vi "Dashboard Main.vi"() -> ()   [LabVIEW 2015]
uses:
  <vilib>/Rock Robotics/WPI/CAN/TalonSRX/WPI_CANTalonSRX_ControlMode.ctl
  <vilib>/Utility/miscctls.llb/LVRowAndColumnTypeDef.ctl
  <vilib>/event_ctls.llb/eventvkey.ctl
  <vilib>/Rock Robotics/WPI/Dashboard/WPI_DashboardLogging Global.vi
  <vilib>/Rock Robotics/Network Tables/NT Read Numeric Array.vi
  <vilib>/Utility/config.llb/Write Key (String).vi
  <vilib>/Utility/config.llb/Write Key (I32).vi
  <vilib>/Utility/config.llb/NI_LVConfig.lvlib
panel:
  in  "Arm State":enum16{"Up", "Down"}(ring)=enum."Down"
  in  "TCP":refnum<k5>
  out "Camera IP":string
  out "Image Message":string="Timeout in Camera Communications"
  in  "Dashboard Tab":T1(tab)
  out "PhotoEye":bool
  in  "Raw Speed":dbl
  out "READY":bool
  out "Shooter Speed":dbl(knob) scale=0.0..100.0
  out "Target Distance":dbl(slide) scale=0.0..30.0
  out "Target Acquired":bool
  in  "Select Auto":string(combo)
  out "NT Connection":bool
  in  "Camera Settings":T2={"Frame Rate"=30, "Compression"=30, "Size"=1} {"Frame Rate" scale=1.0..30.0; "Size" items=["640x480", "320x240", "160x120"]}
  out "MotorChart R":cluster{"Numeric":dbl, "Numeric":dbl}(graph)
  out "MotorChart L":T3(graph)
  out "MotorSliders R":cluster{"MotorSlide1":dbl, "MotorSlide2":dbl} {"MotorSlide2" scale=-1.0..1.0 scale format="%#_2e"; "MotorSlide1" scale=-1.0..1.0 scale format="%#_2e"}
  out "MotorSliders L":T4 {"MotorSlide4 2" scale=0.0..14.0 scale format="%#_2e"; "MotorSlide2" scale=-1.0..1.0 scale format="%#_2e"; "MotorSlide1" scale=-1.0..1.0 scale format="%#_2e"}
  out "JS1 Z":dbl(slide) scale=-1.0..1.0 scale format="%#_2e"
  out "JS1 Graph":cluster{"X":dbl, "Y":dbl}[](graph)
  out "JS1 Buttons":T5
  out "JS2 Z":dbl(slide) scale=-1.0..1.0 scale format="%#_2e"
  out "JS2 Graph":cluster{"X":dbl, "Y":dbl}[](graph)
  out "JS2 Buttons":T5
  out "Mode":T6(ring)=enum."Auto Disabled"
  in  "DB Camera Config":bool
  out "fps":dbl format="%#.1g"
  out "Mbps":dbl format="%#.1g"
  out "Mbps LED":bool
  out "Arm Down":bool
  out "Arm Up":bool
  in  "Vision":u16(ring) items=["Camera Off", "USB Camera SW", "USB Camera HW", "IP Camera"]
  in  "Rec Mode":enum32{"Stop", "Record", "Playback"}(radio)
  out "AUTO 4":bool
  out "AUTO 2":bool
  out "AUTO 1":bool
  out "NO AUTO":bool
  in  "Select Autonomous":u16(knob) scale=0.0..4.0
  out "AUTO 3":bool
  in  "Talon SRX Mode":T7
  in  "Test Slider":dbl(slide) scale=0.0..100.0 scale format="%#_3g"
  in  "On/Off":bool caption="Solenoid"
  in  "Test Name":u16(ring) items=["Select the test to run..."]
  in  "Test Tree":string(tree)
  in  "Motor":cluster{"Value":dbl, "Enable":bool} {"Value" scale=-1.0..1.0 scale format="%#_3g"}
  out "Progress":T8 {"Test Progress" scale=0.0..100.0}
  in  "Rev/Fwd":cluster{"Forward":bool, "Reverse":bool}
  in  "Test Ring":u16(ring) items=["Monochrome", "Color"]
  out "Cmd Status":string
  in  "Execute Command":bool
  in  "Command Params":string[][](table)
  in  "Command Selection":i32(listbox)
  in  "CheckList":i32(listbox)
  out "Tree":string(tree)
  out "Camera Image":T9(plugin-control)
  out "Background":bool
  # "Left"
  # "Front"
  # "Right"
  # "Battery"
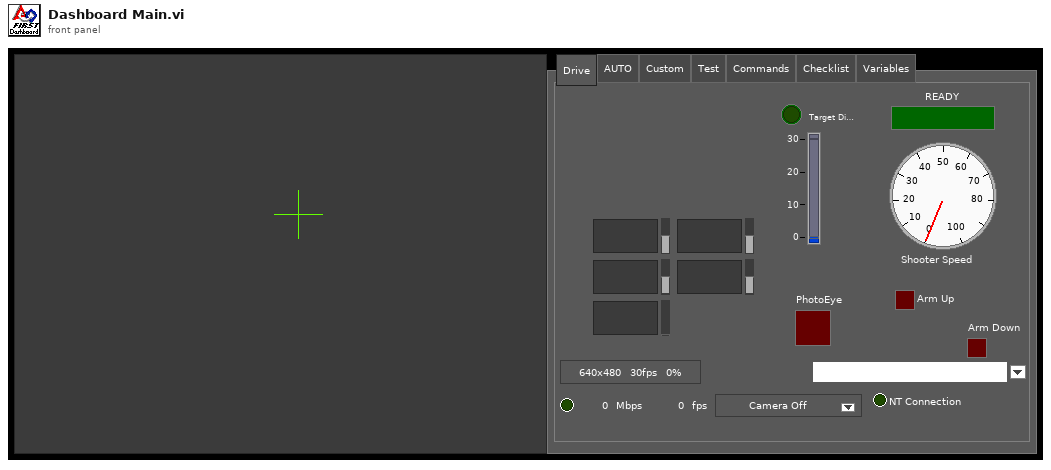
[diagram p1: front panel]
types:
  T1 = enum32{"Drive", "AUTO", "Custom", "Test", "Commands", "Checklist", "Variables"}
  T2 = cluster{"Frame Rate":i32, "Compression":i32, "Size":u16}
  T3 = cluster{"Numeric":dbl, "Numeric":dbl, "Battery V":dbl}
  T4 = cluster{"MotorSlide1":dbl, "MotorSlide2":dbl, "MotorSlide4 2":dbl}
  T5 = cluster{bool, bool, bool, bool, bool, bool, bool, bool, bool, bool, bool, bool}
  T6 = enum8{"Tele-Op Disabled", "Tele-Op Enabled", "Auto Disabled", "Auto Enabled", "Test Disabled", "Test Enabled", "Disconnected", "No Code", "E-Stop"}
  T7 = typedef "WPI_CANTalonSRX_ControlMode.ctl" = enum16{"Throttle (Duty-Cycle)", "Position Closed-Loop", "Velocity Closed-Loop", "Current Closed-Loop", "Voltage Compensation", "Slave Follower", "Motion Profile"}
  T8 = cluster{"Test Progress":u8, "Test Progress Text":string}
  T9 = typedef "IMAQ Image.ctl" = refnum<image>
  T10 = cluster{"IDs":cluster{"RPC field ID":u16, "Unique ID":u16}, "String":string}
  T11 = enum32{"Drive", "Basic", "AUTO", "Test", "Checklist", "Variables"}
  T12 = enum32{"Drive", "Basic", "Custom", "Test", "Checklist", "Variables"}
  T13 = typedef "Image Type" = u32
  T14 = cluster{"Error Strings":string, "Disable Counts":cluster{u16, u16}, "Rail Faults":cluster{u16, u16, u16}, "Robot IP":string, "DB Mode":u8, "Event Info":cluster{"Name":string, "Type":u8, "Number":u16, "Replay":u8}, "Camera Addr":string}
  T15 = cluster{"Storage":cluster{"Disk Free":u64, "RAM Block":u32, "RAM free":u32}, "CPU Utilization":cluster{"CPU % ISR":sgl, "CPU % Time Crit":sgl, "CPU % Timed Str":sgl, "CPU % High":sgl, "CPU % Above":sgl, "CPU % Normal":sgl, "CPU % Low":sgl}, "CAN":cluster{"% Bus Utilization":sgl, "Bus Off Cnt":u32, "TX_FIFO Full Cnt":u32, "Receive Error Cnt":u8, "Transmit Error Cnt":u8}, "HID":cluster{"HID Outputs":u32, "Rumble Low":u16, "Rumble High":u16}[]}
  T16 = cluster{"Status bits":cluster{"Test Mode":bool, "Autonomous":bool, "Enabled":bool, "Code Start":bool, "Brownout":bool, "Reserved 2":bool, "Reserved 3":bool, "E-Stop":bool}, "Code Trace":cluster{"Disabled":bool, "TeleOp":bool, "Auto":bool, "Test":bool}, "Controller Type":enum16{"unknown", "cRIO", "roboRio"}, "Code?":enum16{"unknown", "noCode", "code"}, "Battery V":dbl}
  T17 = cluster{"Control Bits":cluster{"TestMode":bool, "Autonomous":bool, "Enabled":bool, "FMS Present":bool, bool, bool, bool, "E-Stop":bool}, "Team Station ":u8, "Countdown":sgl, "Joystick Values":cluster{"Axes":dbl[], "Buttons":bool[], "POVs":i16[]}[]}
  T18 = cluster{"Axes":dbl[], "Buttons":bool[], "POVs":i16[]}[]
  T19 = cluster{"Axes":dbl[], "Buttons":bool[], "POVs":i16[]}
  T20 = cluster{"Buttons[0]":bool, "Buttons[1]":bool, "Buttons[2]":bool, "Buttons[3]":bool, "Buttons[4]":bool, "Buttons[5]":bool, "Buttons[6]":bool, "Buttons[7]":bool, "Buttons[8]":bool, "Buttons[9]":bool, "Buttons[10]":bool, "Buttons[11]":bool}
  T21 = typedef "NI_LVConfig.lvlib/Config Data RefNum.ctl" = refnum<k1>
  T22 = cluster{"Operation":enum16{"Update", "Clear"}, "Color Box":u32}[]
  T23 = typedef "eventvkey.ctl" = enum16{"ASCII", "Enter", "Return", "Shift", "Ctrl", "Alt", "Cmd", "Opt", "Caps", "NumLock", "Clear", "Break", "Up", "Down", "Left", "Right", "Insert", "Delete", "Home", "End", "PageUp", "PageDown", "Escape", "Help", "Pause", "ScrollLock", "F1", "F2", "F3", "F4", "F5", "F6", "F7", "F8", "F9", "F10", "F11", "F12", "F13", "F14", "F15", "F16", "F17", "F18", "F19", "F20", "F21", "F22", "F23", "F24", "Play", "VolumeUp", "VolumeDown", "Mute", "Two Byte Char"}
  T24 = cluster{"Image Size":bool, "Image Type":bool, "Pixel Value":bool, "ROI Information":bool, "Zoom Factor":bool}
  T25 = enum8{"Enabled", "Disabled", "Disabled and Grayed Out"}
  T26 = cluster{"Operation":enum16{"Update", "Clear"}, "Color Box":u32}
  T27 = typedef "LVRowAndColumnTypeDef.ctl" = cluster{"Row":i32, "Column":i32}
  T28 = cluster{"Shift":bool, "Ctrl":bool, "Alt":bool, "Cmd":bool, "Opt":bool}
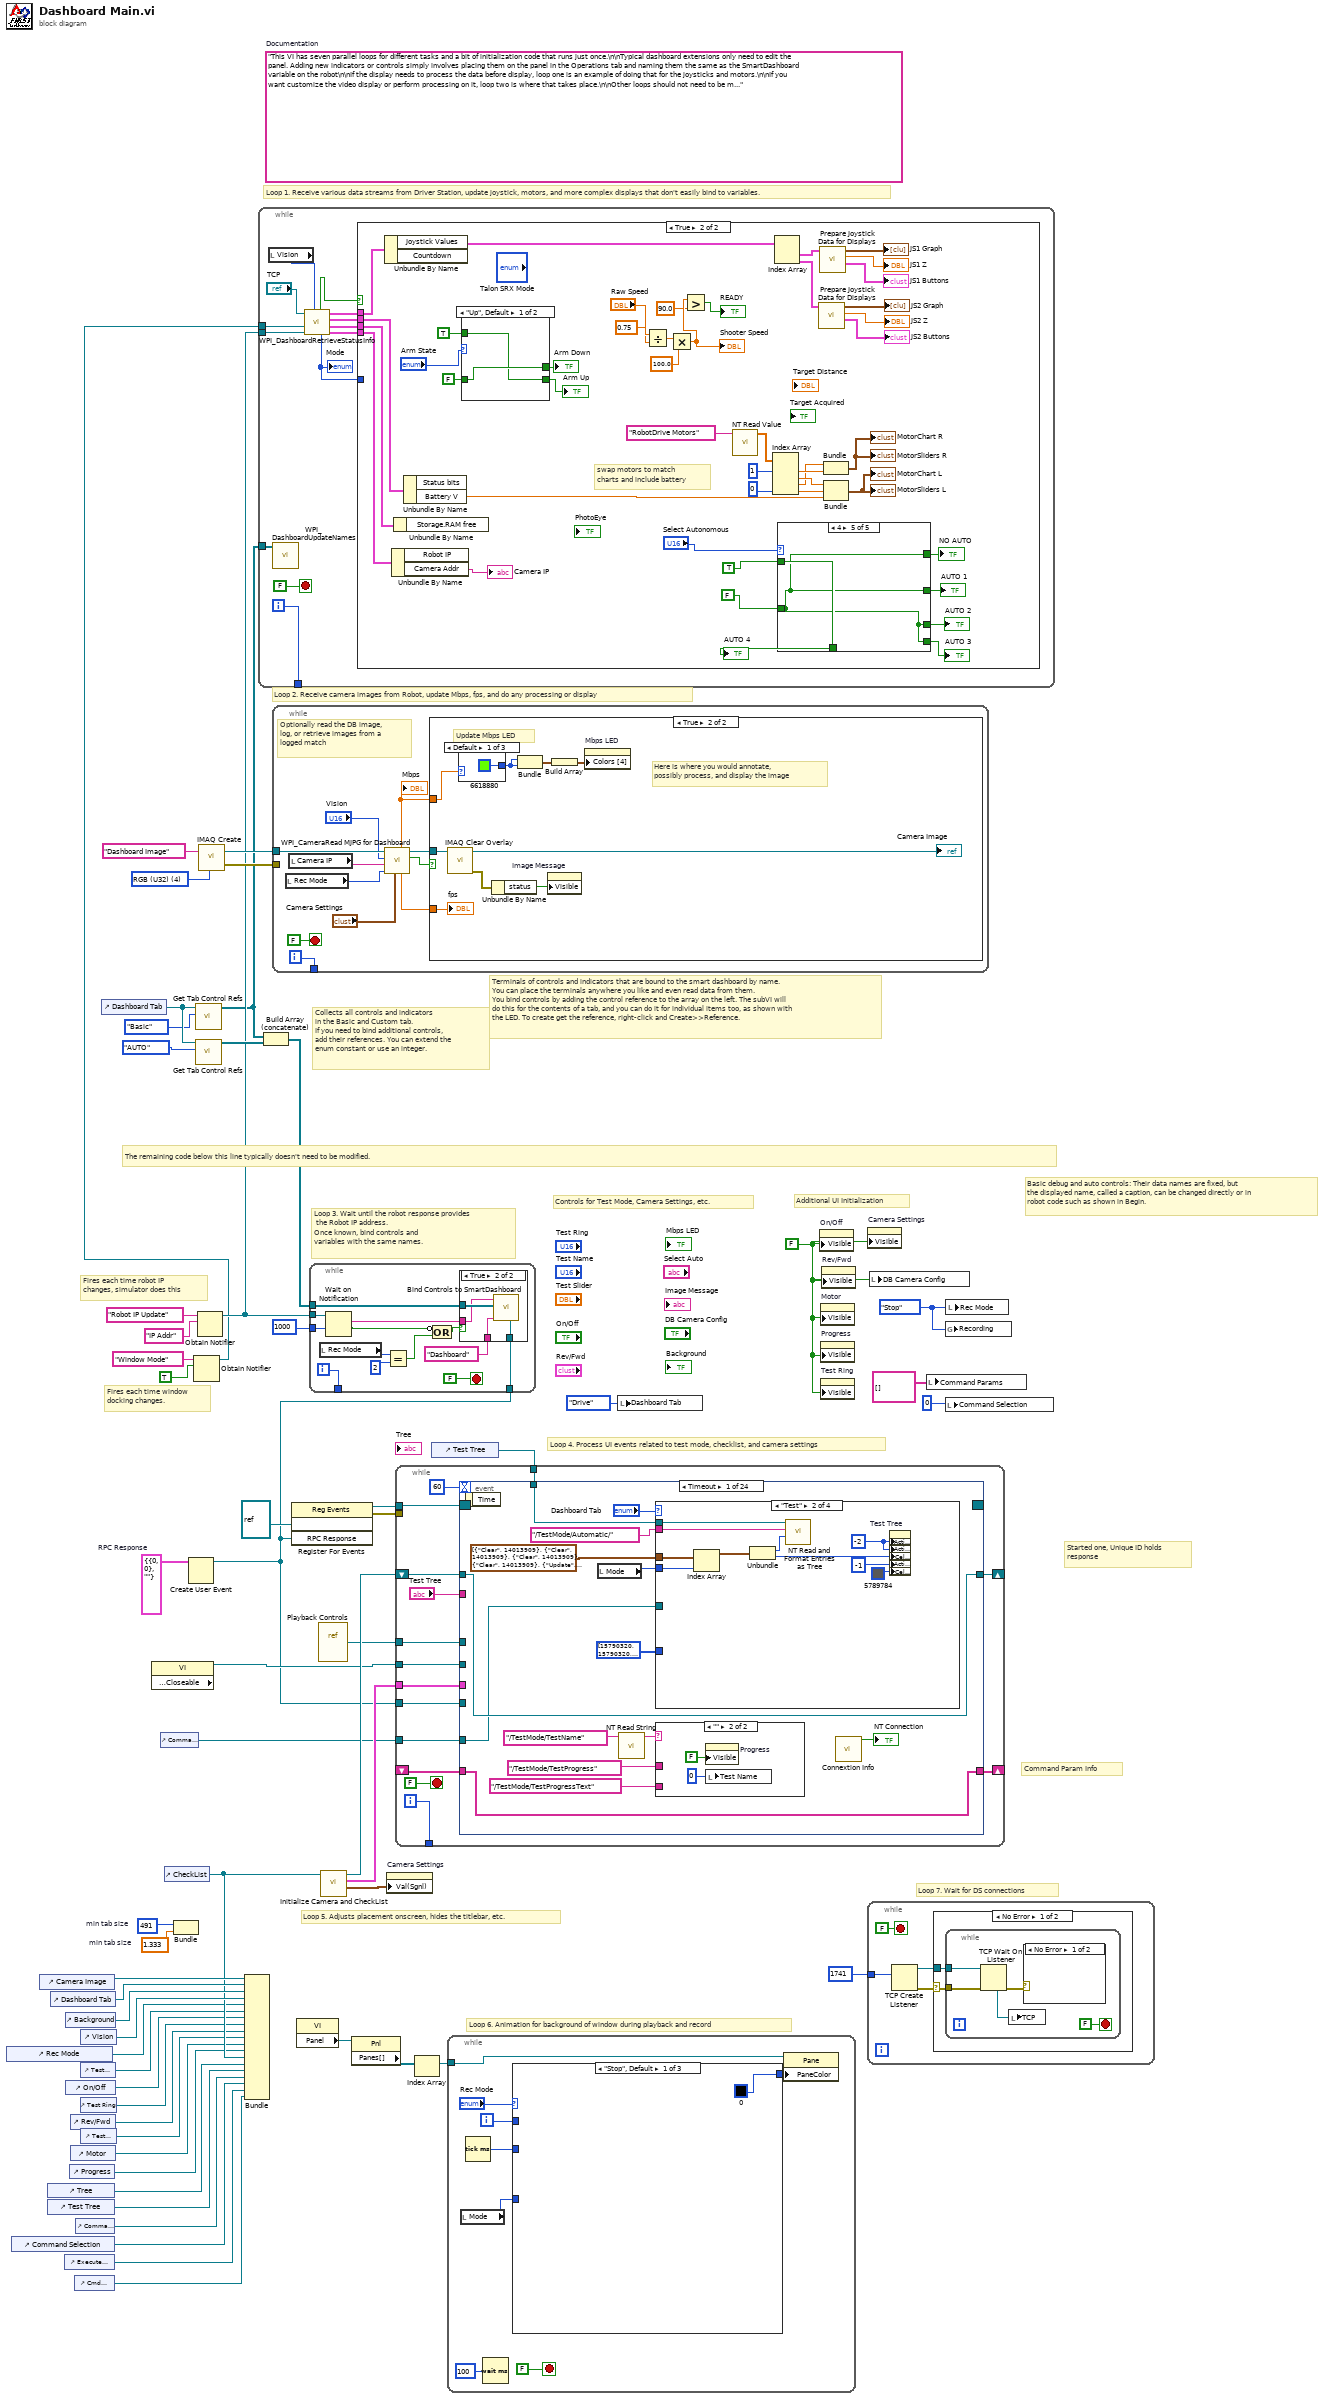
[diagram p0: block diagram]
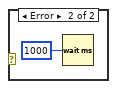
[diagram p2: hidden frame]
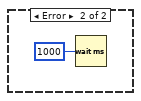
[diagram p3: hidden frame]
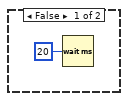
[diagram p4: hidden frame]
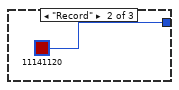
[diagram p10: hidden frame]
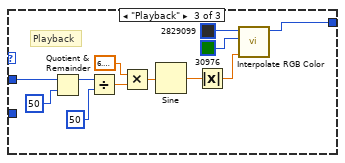
[diagram p11: hidden frame]
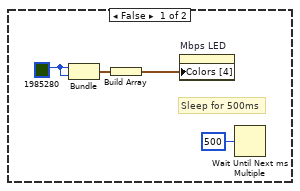
[diagram p13: hidden frame]
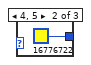
[diagram p14: hidden frame]
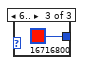
[diagram p15: hidden frame]
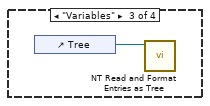
[diagram p17: hidden frame]
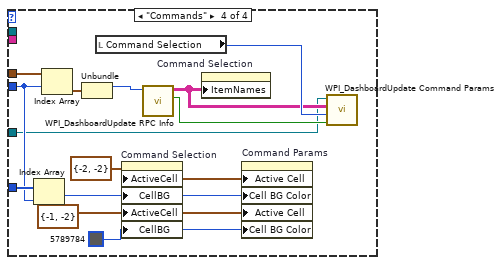
[diagram p18: hidden frame]
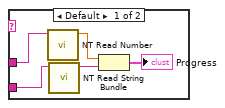
[diagram p19: hidden frame]
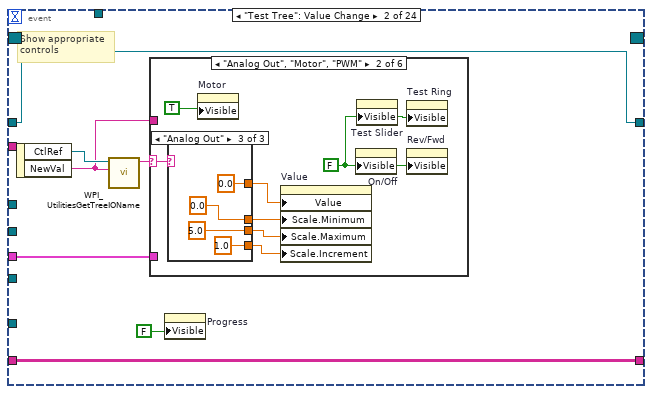
[diagram p20: hidden frame]
diagram:
  w8 = T10 {"IDs"={"RPC field ID"=0, "Unique ID"=0}, "String"=""}  # RPC Response
  w31 = 491  # min tab size
  w30 = 1.333  # min tab size
  w39 = enum32{"Stop", "Record", "Playback"}."Stop" ("Rec Mode")
  w15 = FALSE ("Visible")
  (unwired) "This VI has seven parallel loops for different tasks and a bit of initialization code that runs just once.\n\nTypical dashboard extensions only need to edit the panel. Adding new indicators or controls simply involves placing them on the panel in the Operations tab and naming them the same as the SmartDashboard variable on the robot\n\nIf the display needs to process the data before display, loop one is an example of doing that for the joysticks and motors.\n\nIf you want customize the video display or perform processing on it, loop two is where that takes place.\n\nOther loops should not need to be modified. They are pretty standard, and document the task they perform."  # Documentation
  w59 = T13 4 items=["Grayscale (U8)", "Grayscale (I16)", "Grayscale (SGL)", "Complex (CSG)", "RGB (U32)", "HSL (U32)", "RGB (U64)"] ("Image Type")
  # "Command Param Info"
  # "Started one, Unique ID holds\nresponse"
  # "Loop 7. Wait for DS connections"
  # "Basic debug and auto controls: Their data names are fixed, but\nthe displayed name, called a caption, can be changed directly or in\nrobot code such as shown in Begin."
  # "Controls for Test Mode, Camera Settings, etc."
  # "Additional UI Initialization"
  # "Loop 6. Animation for background of window during playback and record"
  # "Fires each time robot IP\nchanges, simulator does this"
  # "Fires each time window\ndocking changes."
  # "Collects all controls and indicators\nin the Basic and Custom tab.\nIf you need to bind additional controls,\nadd their references. You can extend the\nenum constant or use an integer."
  # "The remaining code below this line typically doesn't need to be modified."
  # "Loop 4. Process UI events related to test mode, checklist, and camera settings"
  # "Terminals of controls and indicators that are bound to the smart dashboard by name.\nYou can place the terminals anywhere you like and even read data from them.\nYou bind controls by adding the control reference to the array on the left. The subVI will\ndo this for the contents of a tab, and you can do it for individual items too, as shown with\nthe LED. To create get the reference, right-click and Create>>Reference."
  # "Loop 3. Wait until the robot response provides\n the Robot IP address.\nOnce known, bind controls and\nvariables with the same names."
  # "Loop 5. Adjusts placement onscreen, hides the titlebar, etc."
  # "Loop 1. Receive various data streams from Driver Station, update joystick, motors, and more complex displays that don't easily bind to variables."
  # "Loop 2. Receive camera images from Robot, update Mbps, fps, and do any processing or display"
  n1 = control-ref of="Rec Mode"() -> (w21:refnum<vi>)
  n2 = control-ref of="Command Selection"() -> (w7:refnum<vi>)
  n3 = control-ref of="Camera Image"() -> (w34:refnum<vi>)
  n4 = control-ref of="Tree"() -> (w25:refnum<vi>)
  n5 = control-ref of="Test Tree"() -> (w24:refnum<vi>)
  n6 = control-ref of="Dashboard Tab"() -> (w33:refnum<vi>)
  n7 = control-ref of="Execute Command"() -> (w9:refnum<vi>)
  n8 = control-ref of="Background"() -> (w29:refnum<vi>)
  n9 = control-ref of="On/Off"() -> (w19:refnum<vi>)
  n10 = control-ref of="Progress"() -> (w16:refnum<vi>)
  n11 = control-ref of="Rev/Fwd"() -> (w17:refnum<vi>)
  n12 = control-ref of="Motor"() -> (w22:refnum<vi>)
  n13 = control-ref of="Cmd Status"() -> (w3:refnum<vi>)
  n14 = control-ref of="Command Params"() -> (w10:refnum<vi>)
  n15 = control-ref of="Test Slider"() -> (w20:refnum<vi>)
  n16 = control-ref of="Vision"() -> (w32:refnum<vi>)
  n17 = control-ref of="Test Ring"() -> (w18:refnum<vi>)
  n18 = control-ref of="Test Name"() -> (w23:refnum<vi>)
  n19 = control-ref of="Dashboard Tab"() -> (w37:refnum<vi>)
  n20 = property class="VI" props=["Front Panel.Closeable"]() -> (reference out=w38:refnum<vi>)  [unwired: 2 in, 2 out]
  n21 = control-ref of="Command Params"() -> (w2:refnum<vi>)
  n22 = control-ref of="CheckList"() -> (w26:refnum<vi>)
  n23 = Bundle("min tab size"=w31, "min tab size"=w30) -> ()  [unwired: 1 in, 1 out]
  n24 = Create User Event(user event datatype=w8) -> (user event=w4:refnum<user-event>)  [unwired: 1 in, 1 out]
  n25 = Obtain Notifier(name (unnamed)="Window Mode", notification data type=TRUE) -> (notifier out=w12:refnum<notifier>)  [unwired: 2 in, 2 out]
  n26 = call <vilib>:"Get Tab Control Refs.vi"("Page Index"=T12."Basic" ("Dashboard Tab"), "TabControl in"=w37) -> ("ControlsOnPage"=w13:refnum<vi>[])  [unwired: 9 in]
  n27 = call <vilib>:"Get Tab Control Refs.vi"("Page Index"=T11."AUTO" ("Dashboard Tab"), "TabControl in"=w37) -> ("ControlsOnPage"=w36:refnum<vi>[])  [unwired: 9 in]
  n28 = Obtain Notifier(name (unnamed)="Robot IP Update", notification data type="IP Addr" ("name (unnamed)")) -> (notifier out=w14:refnum<notifier>)  [unwired: 2 in, 2 out]
  n29 = call "IMAQ Create"("Image Name"="Dashboard Image", "Image Type"=w59) -> ("New Image"=w57:T9, "error out"=w56:errorcluster)  [unwired: 2 in, 1 out]
  n30 = Bundle("Camera Image"=w34, "Dashboard Tab"=w33, "Background"=w29, "Vision"=w32, "Rec Mode"=w21, "Test Slider"=w20, "On/Off"=w19, "Test Ring"=w18, "Rev/Fwd"=w17, "Test Name"=w23, "Motor"=w22, "Progress"=w16, "CheckList"=w26, "Tree"=w25, "Test Tree"=w24, "Command Params"=w10, "Command Selection"=w7, "Execute Command"=w9, "Cmd Status"=w3) -> ()  [unwired: 1 in, 1 out]
  n31 = while {
    tunnel: [w71] -> _
    tunnel: w14 -> [w66]
    tunnel: w13 -> [w65]
    tunnel: w12 -> [w61]
    i -> [w71]
    stop <- FALSE stop-if-true
    n32 = local read "Vision"() -> (w63:u16)
    n33 = call <vilib>:"WPI_DashboardUpdateNames.vi"("Controls on Tab"=w65) -> ()  [unwired: 11 in]
    n34 = call <vilib>:"WPI_DashboardRetrieveStatusInfo.vi"("Vision"=w63, "Binding Refnum"=w66, "Window Mode Notifier"=w61, "TCP Cnx"="TCP") -> ("Power and Errors"=w67:T14, "Robot Metrics"=w69:T15, "Status Info"=w70:T16, "Control Info"=w68:T17, "Robot Mode"=w64:T6, "Process?"=w60:bool)  [unwired: 2 in]
    "Mode" <- w64
    n35 = case shown="True" w60 {
      tunnel: w70 -> [_ w118]
      tunnel: w69 -> [_ w117]
      tunnel: w68 -> [_ w116]
      tunnel: w67 -> [_ w115]
      tunnel: w64 -> [_ _]
      frame False {
        n36 = Wait (ms)(milliseconds to wait=u32 20) -> ()  [unwired: 1 out]
      }
      frame True {
        # "swap motors to match\ncharts and include battery"
        n37 = Unbundle By Name(w116) -> ("Joystick Values"=w105:T18)  [unwired: 1 out]
        n38 = Unbundle By Name(w115) -> ("Camera Addr"=→"Camera IP":string)  [unwired: 1 out]
        n39 = Unbundle By Name(w117) -> ()  [unwired: 1 out]
        n40 = Unbundle By Name(w118) -> ("Battery V"=w106:dbl)  [unwired: 1 out]
        n41 = case shown="\"Up\", Default" "Arm State" {
          tunnel: TRUE -> [w119 w122]
          tunnel: FALSE -> [w120 w121]
          tunnel: [w120 w122] -> w81
          tunnel: [w119 w121] -> w80
          frame "Up", Default {
          }
          frame "Down" {
          }
        }
        "Arm Down" <- w81
        "Arm Up" <- w80
        n42 = Divide(x="Raw Speed", y=0.75) -> (x/y=w91:dbl)
        n43 = Multiply(x=w91, y=100.0) -> (x*y=w88:dbl)
        "Shooter Speed" <- w88
        n44 = Greater?(x=w88, y=90.0) -> (0:→"READY":bool)
        n45 = call-poly <vilib>:"NT Read Value.vi"("Name"="RobotDrive Motors") -> ("Numeric Array"=w94:dbl[])  [unwired: 9 in, 1 out]
        n46 = Index Array(array=w94, index #1=1, index #4=0) -> (element #1=w110:dbl, element #2=w111:dbl, element #3=w109:dbl, element #4=w114:dbl)  [unwired: 2 in]
        n47 = Index Array(array=w105) -> (element #1=w104:T19, element #2=w99:T19)  [unwired: 2 in]
        n48 = case shown="4" "Select Autonomous" {
          tunnel: TRUE -> [w124 w126 w128 w130 w132]
          tunnel: FALSE -> [w123 w125 w127 w129 w131]
          tunnel: [w124 w125 w127 w129 w131] -> w78
          tunnel: [w123 w126 w127 w129 w131] -> w77
          tunnel: [w123 w125 w128 w129 w131] -> w76
          tunnel: [w123 w125 w127 w130 w131] -> w75
          tunnel: [w123 w125 w127 w129 w132] -> w74
          frame 0, Default {
          }
          frame 1 {
          }
          frame 2 {
          }
          frame 3 {
          }
          frame 4 {
          }
        }
        "NO AUTO" <- w78
        "AUTO 1" <- w77
        "AUTO 2" <- w76
        "AUTO 3" <- w75
        "AUTO 4" <- w74
        n49 = call "Prepare Joystick Data for Displays.vi"("Joystick Values"=w99) -> ("Buttons"=→"JS2 Buttons":T20, "Z Axis"=→"JS2 Z":dbl, "Cartesian Data"=→"JS2 Graph":cluster{"X axis":dbl, "X axis":dbl}[])  [unwired: 8 in]
        n50 = call "Prepare Joystick Data for Displays.vi"("Joystick Values"=w104) -> ("Buttons"=→"JS1 Buttons":T20, "Z Axis"=→"JS1 Z":dbl, "Cartesian Data"=→"JS1 Graph":cluster{"X axis":dbl, "X axis":dbl}[])  [unwired: 8 in]
        n51 = Bundle("Numeric"=w109, "Numeric"=w110) -> (→"MotorChart R" →"MotorSliders R":cluster{"Numeric":dbl, "Numeric":dbl})  [unwired: 1 in]
        n52 = Bundle("Numeric"=w111, "Numeric"=w114, "Battery V"=w106) -> (→"MotorChart L" →"MotorSliders L":T3)  [unwired: 1 in]
      }
    }
  }
  n53 = Build Array (concatenate)(w13, w36) -> (w35:refnum<vi>[])
  n54 = while {
    tunnel: w57 -> [w141]
    tunnel: w56 -> [_]
    tunnel: [w142] -> _
    i -> [w142]
    stop <- FALSE stop-if-true
    # "Optionally read the DB image,\nlog, or retrieve images from a\nlogged match"
    n55 = local read "Rec Mode"() -> (w136:enum32{"Stop", "Record", "Playback"})
    n56 = local read "Camera IP"() -> (w134:string)
    n57 = call <vilib>:"WPI_CameraRead MJPG for Dashboard.vi"("Camera Settings"="Camera Settings", "Rec Mode"=w136, "Camera IP"=w134, "Camera Mode"="Vision", "Refnum in"=w141) -> ("Active"=w139:bool, "Refnum out"=w140:T9, "FPS"=w138:dbl, "Bandwidth (Mbps)"=w133:dbl)  [unwired: 3 in]
    "Mbps" <- w133
    n58 = case shown="True" w139 {
      tunnel: w140 -> [_ w151]
      tunnel: w133 -> [_ w150]
      tunnel: w138 -> [_ w148]
      frame False {
        w144 = u32 1985280 ("Color Box")
        # "Sleep for 500ms"
        n59 = Bundle("Color Box"=w144, "Color Box"=w144) -> (w146:cluster{"Color Box":u32, "Color Box":u32})  [unwired: 1 out]
        n60 = Build Array(w146) -> (w145:cluster{"Color Box":u32, "Color Box":u32}[])
        n61 = property on="Mbps LED" class="Bool (strict)"("Colors [4]"=w145) -> ()  [unwired: 2 in, 2 out]
        n62 = Wait Until Next ms Multiple(millisecond multiple=u32 500) -> ()  [unwired: 1 out]
      }
      frame True {
        # "Here is where you would annotate,\npossibly process, and display the image"
        # "Update Mbps LED"
        n63 = call "IMAQ Clear Overlay"("Image"=w151) -> ("error out"=w155:errorcluster, "Image Out"=→"Camera Image":T9)  [unwired: 2 in, 7 out]
        n64 = case shown="Default" w150 {
          tunnel: [u32 6618880 ("Color Box") u32 16776722 ("Color Box") u32 16716800 ("Color Box")] -> w152
          frame Default {
          }
          frame 4, 5 {
          }
          frame 6.. {
          }
        }
        n65 = Unbundle By Name(w155) -> ("status"=w156:bool)
        n66 = Bundle("Color Box"=w152, "Color Box"=w152) -> (w154:cluster{"Color Box":u32, "Color Box":u32})  [unwired: 1 out]
        n67 = property on="Image Message" class="Str"("Visible"=w156) -> ()  [unwired: 2 in, 2 out]
        n68 = Build Array(w154) -> (w153:cluster{"Color Box":u32, "Color Box":u32}[])
        n69 = property on="Mbps LED" class="Bool (strict)"("Colors [4]"=w153) -> ()  [unwired: 2 in, 2 out]
        "fps" <- w148
      }
    }
  }
  n70 = register-events(refnum<vi> refnum, w4) -> (reference out=w43:refnum<event-registration>, error out=w42:errorcluster)  [unwired: 2 in]
  n71 = property class="VI"() -> ("Panel"=w46:refnum<vi>)  [unwired: 2 in, 2 out]
  n72 = while {
    tunnel: w35 -> [w172]
    tunnel: w14 -> [w170]
    tunnel: [w168] -> _
    tunnel: u32 1000 ("milliseconds to wait") -> [w167]
    tunnel: w4 -> [w160]
    i -> [w168]
    stop <- FALSE stop-if-true
    n73 = local read "Rec Mode"() -> (w163:enum32{"Stop", "Record", "Playback"})
    n74 = Wait on Notification(notifier=w170, timeout in ms (-1)=w167) -> (notification=w169:string, timed out?=w165:bool)  [unwired: 2 in, 2 out]
    n75 = Equal?(x=w163, y=u16 2 ("Rec Mode")) -> (x = y?=w164:bool)
    n76 = Compound Arithmetic op=OR(invert w165, w164) -> (w166:bool)
    n77 = case shown="True" w166 {
      tunnel: w172 -> [_ w176]
      tunnel: w169 -> [_ w175]
      tunnel: "Dashboard" -> [_ w174]
      tunnel: w160 -> [_ w173]
      frame False {
      }
      frame True {
        n78 = call <vilib>:"Bind Controls to SmartDashboard.vi"("RPC ref"=w173, "Client Name"=w174, "Bound Control Refs"=w176, "Server IP Address"=w175) -> ()  [unwired: 8 in]
      }
    }
  }
  n79 = vi-ref "Playback Controls.vi"() -> (w44:refnum<vi>)
  n80 = call "Initialize Camera and CheckList.vi"("ListBox in"=w26) -> ("Cluster"=w50:cluster{"value":i32, "value":i32, "index":i32}, "Array"=w51:cluster{string[]}[], "File Refnum"=w49:T21)  [unwired: 8 in]
  n81 = property class="Pnl"(reference=w46) -> ("Panes[]"=w47:refnum<vi>[])  [unwired: 1 in, 2 out]
  n82 = property on="Camera Settings" class="Clust (strict)"("Val(Sgnl)"=w50) -> ()  [unwired: 2 in, 2 out]
  n83 = Index Array(array=w47) -> (element=w45:refnum<vi>)  [unwired: 1 in]
  n84 = control-ref of="Test Tree"() -> (w48:refnum<vi>)
  n85 = while {
    tunnel: w51 -> [w188]
    shift-right: [w187] -> _
    shift-left: w49 -> [w186]
    tunnel: [w185] -> _
    tunnel: w48 -> [w184]
    tunnel: w44 -> [w183]
    tunnel: w43 -> [w182]
    tunnel: w42 -> [_]
    tunnel: w38 -> [w181]
    tunnel: w4 -> [w180]
    tunnel: w2 -> [w179]
    shift-right: [w178] -> _
    shift-left: _ -> [w177]
    i -> [w185]
    stop <- FALSE stop-if-true
    n86 = event shown="[0] Timeout" {
      selector: w182 -> [_ _ _ _ _ _ _ _ _ _ _ _ _ _ _ _ _ _ _ _ _ _ _ _]
      dyn-events: [_ _ _ _ _ _ _ _ _ _ _ _ _ _ _ _ _ _ w497 _ _ _ _ _] -> _
      timeout: u32 60 ("milliseconds to wait") -> [_ _ _ _ _ _ _ _ _ _ _ _ _ _ _ _ _ _ _ _ _ _ _ _]
      tunnel: w184 -> [w201 _ _ _ _ _ _ _ _ _ _ _ _ _ _ _ _ _ _ _ _ _ _ _]
      tunnel: "Test Tree" -> [_ _ _ _ _ _ _ _ _ _ _ _ _ w460 w469 w472 w477 w486 _ _ _ _ _ _]
      tunnel: w188 -> [_ w239 _ _ _ _ _ _ _ _ _ w422 w453 _ _ _ _ _ _ _ _ _ _ _]
      tunnel: [w198 w238 w342 w348 w358 w362 w368 w380 w388 w394 w407 w421 w446 w459 w467 w471 w476 w485 w499 w515 w517 w525 w536 w541] -> w187
      tunnel: w186 -> [w198 w238 w342 w348 w358 w362 w368 w380 w388 w394 w407 w420 w446 w459 w467 w471 w476 w485 w499 w515 w517 w525 w536 w541]
      tunnel: w183 -> [_ _ _ _ _ _ _ _ _ _ _ _ _ _ _ _ _ _ w500 _ w520 _ _ _]
      tunnel: w181 -> [_ _ _ _ _ _ _ _ _ _ _ _ _ _ _ _ _ _ w495 _ _ _ _ _]
      tunnel: w180 -> [_ _ _ _ _ _ _ _ _ _ _ _ _ _ _ _ _ _ w491 _ _ _ _ _]
      tunnel: w179 -> [w193 _ _ _ _ _ w366 _ _ _ _ _ _ _ _ _ _ _ _ _ _ _ _ _]
      tunnel: [w192 w237 w341 w347 w357 w363 w364 w374 w385 w393 w406 w419 w445 w458 w466 w470 w475 w484 w490 w513 w516 w521 w529 w542] -> w178
      tunnel: w177 -> [w192 w237 w341 w347 w357 w363 w364 _ _ w393 w406 w419 w445 w458 w466 w470 w475 w484 w490 w513 w516 w521 w529 w542]
      event Timeout {
        n87 = event-data() -> ()  [unwired: 1 in, 1 out]
        n88 = local read "Mode"() -> (w195:T6)
        n89 = call <vilib>:"NT Read String.vi"("Name"="/TestMode/TestName") -> ("String"=w204:string)  [unwired: 9 in, 1 out]
        n90 = case shown="\"Test\"" "Dashboard Tab" {
          tunnel: w201 -> [_ w215 _ _]
          tunnel: "/TestMode/Automatic/" ("Name Pattern") -> [_ w214 _ _]
          tunnel: T22 [{"Operation"=enum."Clear", "Color Box"=14013909}, {"Operation"=enum."Clear", "Color Box"=14013909}, {"Operation"=enum."Clear", "Color Box"=14013909}, {"Operation"=enum."Clear", "Color Box"=14013909}, {"Operation"=enum."Update", "Color Box"=14013909}, {"Operation"=enum."Update", "Color Box"=16777215}, {"Operation"=enum."Clear", "Color Box"=14013909}, {"Operation"=enum."Clear", "Color Box"=14013909}, {"Operation"=enum."Clear", "Color Box"=14013909}] -> [_ w207 _ w224]
          tunnel: w195 -> [_ w206 _ w223]
          tunnel: u32[] [15790320, 15790320, 15790320, 15790320, 16777215, 16777215, 15790320, 15790320, 15790320] -> [_ _ _ w229]
          tunnel: w193 -> [_ _ _ w217]
          frame "Custom", Default {
          }
          frame "Test" {
            w213 = -2 ("Active Item:Row Number")
            n91 = Index Array(array=w207, index=w206) -> (element=w208:T26)
            n92 = Unbundle(w208) -> ("Operation"=w209:enum16{"Update", "Clear"}, "Color Box"=w210:u32)
            n93 = call <vilib>:"NT Read and Format Entries as Tree.vi"("Operation"=w209, "Name Pattern"=w214, "Tree Refnum"=w215) -> ()  [unwired: 7 in, 2 out]
            n94 = property on="Test Tree" class="Tree (strict)"("Active Item Row Number"=w213, "ActiveColNum"=w213, "CellBG"=w210, "Active Item Row Number"=-1 ("Active Item:Row Number"), "CellBG"=u32 5789784 ("Color Box")) -> ()  [unwired: 2 in, 2 out]
          }
          frame "Variables" {
            n95 = control-ref of="Tree"() -> (w216:refnum<vi>)
            n96 = call <vilib>:"NT Read and Format Entries as Tree.vi"("Tree Refnum"=w216) -> ()  [unwired: 9 in, 2 out]
          }
          frame "Commands" {
            w225 = u32 5789784 ("Color Box")
            w226 = T27 {"Row"=-1, "Column"=-2} ("Active Cell:Active Cell")
            w228 = T27 {"Row"=-2, "Column"=-2} ("Active Cell:Active Cell")
            n97 = Index Array(array=w229, index=w223) -> (element=w227:u32)
            n98 = Index Array(array=w224, index=w223) -> (element=w222:T26)
            n99 = Unbundle(w222) -> ("Operation"=w221:enum16{"Update", "Clear"})  [unwired: 1 out]
            n100 = local read "Command Selection"() -> (w220:i32)
            n101 = property on="Command Selection" class="MCListbox (strict)"("ActiveCell"=w228, "CellBG"=w227, "ActiveCell"=w226, "CellBG"=w225) -> ()  [unwired: 2 in, 2 out]
            n102 = call <vilib>:"WPI_DashboardUpdate RPC Info.vi"("Operation"=w221) -> ("update"=w219:bool, "commands"=w218:string[][])  [unwired: 9 in]
            n103 = property on="Command Selection" class="MCListbox (strict)"("ItemNames"=w218) -> ()  [unwired: 2 in, 2 out]
            n104 = property on="Command Params" class="Tbl (strict)"("Active Cell"=w228, "Cell BG Color"=w227, "Active Cell"=w226, "Cell BG Color"=w225) -> ()  [unwired: 2 in, 2 out]
            n105 = call <vilib>:"WPI_DashboardUpdate Command Params.vi"("Update"=w219, "NewVal"=w220, "Commands"=w218, "Param Tbl"=w217) -> ()  [unwired: 7 in, 1 out]
          }
        }
        n106 = case shown="\"\"" w204 {
          tunnel: "/TestMode/TestProgress" ("Name") -> [w231 _]
          tunnel: "/TestMode/TestProgressText" ("Name") -> [w230 _]
          frame Default {
            n107 = call <vilib>:"NT Read Number.vi"("Name"=w231) -> ("Numeric"=w232:dbl)  [unwired: 9 in, 1 out]
            n108 = call <vilib>:"NT Read String.vi"("Name"=w230) -> ("String"=w233:string)  [unwired: 9 in, 1 out]
            n109 = Bundle("Numeric"=w232, "String"=w233) -> (→"Progress":cluster{"Numeric":dbl, "String":string})  [unwired: 1 in]
          }
          frame "" {
            n110 = property on="Progress" class="Clust (strict)"("Visible"=FALSE) -> ()  [unwired: 2 in, 2 out]
            n111 = local write "Test Name"(u16 0) -> ()
          }
        }
        n112 = call <vilib>:"Connextion Info.vi"() -> ("Connected"=→"NT Connection":bool)  [unwired: 10 in, 1 out]
      }
      event "Test Tree": Value Change {
        # "Show appropriate\ncontrols"
        n113 = event-data() -> ("CtlRef"=w242:refnum<vi>, "NewVal"=w240:string)  [unwired: 1 in]
        n114 = call <vilib>:"WPI_UtilitiesGetTreeIOName.vi"("NewVal"=w240, "TreeControl in"=w242) -> ("I/O Name"=w243:string)  [unwired: 9 in]
        n115 = case shown="\"Analog Out\", \"Motor\", \"PWM\"" w243 {
          selector: w243 -> [_ w250 _ w272 w281 _]
          tunnel: w240 -> [_ _ w269 w271 _ w288]
          tunnel: w239 -> [_ _ _ _ _ w287]
          frame Default {
            w245 = FALSE ("Visible")
            w244 = FALSE ("Visible")
            n116 = property on="Motor" class="Clust (strict)"("Visible"=w244) -> ()  [unwired: 2 in, 2 out]
            n117 = property on="Test Ring" class="Ring (strict)"("Visible"=w244) -> ()  [unwired: 2 in, 2 out]
            n118 = property on="Rev/Fwd" class="Clust (strict)"("Visible"=w245) -> ()  [unwired: 2 in, 2 out]
            n119 = property on="On/Off" class="Bool (strict)"("Visible"=w245) -> ()  [unwired: 2 in, 2 out]
            n120 = property on="Test Slider" class="Slide (strict)"("Visible"=w245) -> ()  [unwired: 2 in, 2 out]
          }
          frame "Analog Out", "Motor", "PWM" {
            w251 = FALSE ("Visible")
            n121 = case shown="\"Analog Out\"" w250 {
              tunnel: [1.0 ("Value") -1.0 ("Value") 0.0 ("Value")] -> w249
              tunnel: [255.0 ("Value") 1.0 ("Value") 5.0 ("Value")] -> w248
              tunnel: [128.0 ("Value") 0.0 ("Value") 0.0 ("Value")] -> w247
              tunnel: [64.0 ("Value") 0.5 ("Value") 1.0 ("Value")] -> w246
              frame "PWM" {
              }
              frame "Motor", Default {
              }
              frame "Analog Out" {
              }
            }
            n122 = property on="Motor" class="Clust (strict)"("Visible"=TRUE) -> ()  [unwired: 2 in, 2 out]
            n123 = property on="Value" class="Slide (strict)"("Value"=w247, "Scale.Minimum"=w249, "Scale.Maximum"=w248, "Scale.Increment"=w246) -> ()  [unwired: 2 in, 2 out]
            n124 = property on="On/Off" class="Bool (strict)"("Visible"=w251) -> ()  [unwired: 2 in, 2 out]
            n125 = property on="Test Slider" class="Slide (strict)"("Visible"=w251) -> ()  [unwired: 2 in, 2 out]
            n126 = property on="Test Ring" class="Ring (strict)"("Visible"=w251) -> ()  [unwired: 2 in, 2 out]
            n127 = property on="Rev/Fwd" class="Clust (strict)"("Visible"=w251) -> ()  [unwired: 2 in, 2 out]
          }
          frame "Servo" {
            w267 = FALSE ("Visible")
            n128 = call <vilib>:"NT Read Number.vi"("Name"=w269) -> ("Numeric"=w268:dbl)  [unwired: 9 in, 1 out]
            n129 = property on="Test Slider" class="Slide (strict)"("Visible"=TRUE, "Scale.Maximum"=170.0 ("Scale.Range:Maximum")) -> ()  [unwired: 2 in, 2 out]
            n130 = local write "Test Slider"(w268) -> ()
            n131 = property on="Motor" class="Clust (strict)"("Visible"=w267) -> ()  [unwired: 2 in, 2 out]
            n132 = property on="Rev/Fwd" class="Clust (strict)"("Visible"=w267) -> ()  [unwired: 2 in, 2 out]
            n133 = property on="On/Off" class="Bool (strict)"("Visible"=w267) -> ()  [unwired: 2 in, 2 out]
            n134 = property on="Test Ring" class="Ring (strict)"("Visible"=w267) -> ()  [unwired: 2 in, 2 out]
          }
          frame "Relay", "Solenoid" {
            w270 = FALSE ("Visible")
            n135 = property on="Motor" class="Clust (strict)"("Visible"=w270) -> ()  [unwired: 2 in, 2 out]
            n136 = property on="Test Slider" class="Slide (strict)"("Visible"=w270) -> ()  [unwired: 2 in, 2 out]
            n137 = Search and Replace String(input string=w271, search string="/Value  **", replace string="/Direction") -> (result string=w277:string)  [unwired: 5 in, 3 out]
            n138 = property on="Test Ring" class="Ring (strict)"("Visible"=w270) -> ()  [unwired: 2 in, 2 out]
            n139 = call <vilib>:"NT Read String.vi"("Name"=w277) -> ("String"=w275:string)  [unwired: 9 in, 1 out]
            n140 = Equal?(x="Both directions", y=w275) -> (x = y?=w273:bool)
            n141 = Not(x=w273) -> (.not. x?=w274:bool)
            n142 = property on="Rev/Fwd" class="Clust (strict)"("Visible"=w273) -> ()  [unwired: 2 in, 2 out]
            n143 = property on="On/Off" class="Bool (strict)"("Visible"=w274, "Caption.Text"=w272) -> ()  [unwired: 2 in, 2 out]
          }
          frame "Compressor", "Digital Out" {
            w280 = FALSE ("Visible")
            # "Get direction and finish"
            n144 = property on="Motor" class="Clust (strict)"("Visible"=w280) -> ()  [unwired: 2 in, 2 out]
            n145 = property on="Test Slider" class="Slide (strict)"("Visible"=w280) -> ()  [unwired: 2 in, 2 out]
            n146 = property on="Test Ring" class="Ring (strict)"("Visible"=w280) -> ()  [unwired: 2 in, 2 out]
            n147 = property on="On/Off" class="Bool (strict)"("Visible"=TRUE, "Caption.Text"=w281) -> ()  [unwired: 2 in, 2 out]
            n148 = property on="Rev/Fwd" class="Clust (strict)"("Visible"=FALSE) -> ()  [unwired: 2 in, 2 out]
          }
          frame "Camera" {
            n149 = call <vilib>:"Get Last Path Segment.vi"("String in"=w288) -> ("String out"=w289:string)  [unwired: 10 in]
            n150 = property on="On/Off" class="Bool (strict)"("Visible"=FALSE) -> ()  [unwired: 2 in, 2 out]
            n151 = property on="Motor" class="Clust (strict)"("Visible"=FALSE) -> ()  [unwired: 2 in, 2 out]
            n152 = property on="Rev/Fwd" class="Clust (strict)"("Visible"=FALSE) -> ()  [unwired: 2 in, 2 out]
            n153 = case shown="\"White Balance  **\"" w289 {
              tunnel: w288 -> [w295 w304 w313 w322 w331 _ w337]
              tunnel: w287 -> [w293 w301 w310 w319 w328 _ _]
              frame "Size  **" {
                n154 = Index Array(array=w293) -> (element=w292:cluster{string[]})  [unwired: 1 in]
                n155 = call <vilib>:"NT Read String.vi"("Name"=w295) -> ("String"=w294:string)  [unwired: 9 in, 1 out]
                n156 = Unbundle(w292) -> (w290:string[])
                n157 = Match First String(2:w290, 3:w294) -> (0:w291:i32)  [unwired: 1 out]
                n158 = property on="Test Ring" class="Ring (strict)"("Value"=w291, "Strings []"=w290) -> ()  [unwired: 2 in, 2 out]
                n159 = property on="Test Ring" class="Ring (strict)"("Visible"=TRUE) -> ()  [unwired: 2 in, 2 out]
                n160 = property on="Test Slider" class="Slide (strict)"("Visible"=FALSE) -> ()  [unwired: 2 in, 2 out]
              }
              frame "White Balance  **" {
                n161 = Index Array(array=w301, index=1) -> (element=w302:cluster{string[]})
                n162 = call <vilib>:"NT Read String.vi"("Name"=w304) -> ("String"=w303:string)  [unwired: 9 in, 1 out]
                n163 = Unbundle(w302) -> (w299:string[])
                n164 = Match First String(2:w299, 3:w303) -> (0:w298:i32)  [unwired: 1 out]
                n165 = property on="Test Ring" class="Ring (strict)"("Value"=w298, "Strings []"=w299) -> ()  [unwired: 2 in, 2 out]
                n166 = property on="Test Ring" class="Ring (strict)"("Visible"=TRUE) -> ()  [unwired: 2 in, 2 out]
                n167 = property on="Test Slider" class="Slide (strict)"("Visible"=FALSE) -> ()  [unwired: 2 in, 2 out]
              }
              frame "Exposure  **" {
                n168 = Index Array(array=w310, index=2) -> (element=w311:cluster{string[]})
                n169 = call <vilib>:"NT Read String.vi"("Name"=w313) -> ("String"=w312:string)  [unwired: 9 in, 1 out]
                n170 = Unbundle(w311) -> (w307:string[])
                n171 = Match First String(2:w307, 3:w312) -> (0:w308:i32)  [unwired: 1 out]
                n172 = property on="Test Ring" class="Ring (strict)"("Value"=w308, "Strings []"=w307) -> ()  [unwired: 2 in, 2 out]
                n173 = property on="Test Ring" class="Ring (strict)"("Visible"=TRUE) -> ()  [unwired: 2 in, 2 out]
                n174 = property on="Test Slider" class="Slide (strict)"("Visible"=FALSE) -> ()  [unwired: 2 in, 2 out]
              }
              frame "Exposure Priority  **" {
                n175 = Index Array(array=w319, index=3) -> (element=w320:cluster{string[]})
                n176 = call <vilib>:"NT Read String.vi"("Name"=w322) -> ("String"=w321:string)  [unwired: 9 in, 1 out]
                n177 = Unbundle(w320) -> (w316:string[])
                n178 = Match First String(2:w316, 3:w321) -> (0:w317:i32)  [unwired: 1 out]
                n179 = property on="Test Ring" class="Ring (strict)"("Value"=w317, "Strings []"=w316) -> ()  [unwired: 2 in, 2 out]
                n180 = property on="Test Ring" class="Ring (strict)"("Visible"=TRUE) -> ()  [unwired: 2 in, 2 out]
                n181 = property on="Test Slider" class="Slide (strict)"("Visible"=FALSE) -> ()  [unwired: 2 in, 2 out]
              }
              frame "Color Enable  **" {
                n182 = Index Array(array=w328, index=4) -> (element=w329:cluster{string[]})
                n183 = call <vilib>:"NT Read String.vi"("Name"=w331) -> ("String"=w330:string)  [unwired: 9 in, 1 out]
                n184 = Unbundle(w329) -> (w325:string[])
                n185 = Match First String(2:w325, 3:w330) -> (0:w326:i32)  [unwired: 1 out]
                n186 = property on="Test Ring" class="Ring (strict)"("Value"=w326, "Strings []"=w325) -> ()  [unwired: 2 in, 2 out]
                n187 = property on="Test Ring" class="Ring (strict)"("Visible"=TRUE) -> ()  [unwired: 2 in, 2 out]
                n188 = property on="Test Slider" class="Slide (strict)"("Visible"=FALSE) -> ()  [unwired: 2 in, 2 out]
              }
              frame Default {
                n189 = property on="Test Ring" class="Ring (strict)"("Visible"=FALSE) -> ()  [unwired: 2 in, 2 out]
                n190 = property on="Test Slider" class="Slide (strict)"("Visible"=FALSE) -> ()  [unwired: 2 in, 2 out]
              }
              frame "Brightness  **", "Color Level  **", "Compression  **", "FPS  **", "Sharpness  **" {
                n191 = call <vilib>:"NT Read Number.vi"("Name"=w337) -> ("Numeric"=w336:dbl)  [unwired: 9 in, 1 out]
                n192 = local write "Test Slider"(w336) -> ()
                n193 = property on="Test Slider" class="Slide (strict)"("Visible"=TRUE, "Scale.Maximum"=100.0 ("Scale.Range:Maximum")) -> ()  [unwired: 2 in, 2 out]
                n194 = property on="Test Ring" class="Ring (strict)"("Visible"=FALSE) -> ()  [unwired: 2 in, 2 out]
              }
            }
          }
        }
        n195 = property on="Progress" class="Clust (strict)"("Visible"=FALSE) -> ()  [unwired: 2 in, 2 out]
      }
      event "Test Name": Mouse Enter {
        # "Populate the ring with the list of tests"
        n196 = event-data() -> ()  [unwired: 1 in, 1 out]
        n197 = call <vilib>:"NT Read String Array.vi"("Name"="/TestMode/TestList") -> ("String Array"=w346:string[])  [unwired: 9 in, 1 out]
        n198 = Build Array (concatenate)("Select the test to run...", w346) -> (w345:string[])
        n199 = property on="Test Name" class="Ring (strict)"("Strings []"=w345) -> ()  [unwired: 2 in, 2 out]
      }
      event "Test Name": Value Change {
        w349 = FALSE ("Visible")
        # "Tell the robot the test name to run"
        n200 = event-data() -> ("NewVal"=w353:u16)  [unwired: 1 in]
        n201 = property on="Test Name" class="Ring (strict)"() -> ("Strings []"=w354:string[])  [unwired: 2 in, 2 out]
        n202 = local write "Progress"(T8 {"Test Progress"=0, "Test Progress Text"=""} ("Progress")) -> ()
        n203 = Index Array(array=w354, index=w353) -> (element=w352:string)
        n204 = call <vilib>:"NT Write String.vi"("String"=w352, "Name"="/TestMode/TestName") -> ()  [unwired: 9 in, 1 out]
        n205 = property on="Progress" class="Clust (strict)"("Visible"=TRUE) -> ()  [unwired: 2 in, 2 out]
        n206 = property on="Motor" class="Clust (strict)"("Visible"=w349) -> ()  [unwired: 2 in, 2 out]
        n207 = property on="Test Slider" class="Slide (strict)"("Visible"=w349) -> ()  [unwired: 2 in, 2 out]
        n208 = property on="On/Off" class="Bool (strict)"("Visible"=w349) -> ()  [unwired: 2 in, 2 out]
        n209 = property on="Rev/Fwd" class="Clust (strict)"("Visible"=w349) -> ()  [unwired: 2 in, 2 out]
        n210 = property on="Test Ring" class="Ring (strict)"("Visible"=w349) -> ()  [unwired: 2 in, 2 out]
      }
      event "Select Auto": Mouse Enter {
        # "Populate the combo box with the list of autonomous options"
        n211 = event-data() -> ()  [unwired: 1 in, 1 out]
        n212 = call <vilib>:"NT Read String Array.vi"("Name"="Auto List") -> ("String Array"=w356:string[])  [unwired: 9 in, 1 out]
        n213 = property on="Select Auto" class="CmbBox"("Strings[]"=w356) -> ()  [unwired: 2 in, 2 out]
      }
      event "Select Auto": Value Change {
        # "User modified the Auto Selection. Write to NT variable so robot knows."
        n214 = event-data() -> ("NewVal"=w360:string)  [unwired: 1 in]
        n215 = call <vilib>:"NT Write String.vi"("String"=w360, "Name"="Auto Selector") -> ()  [unwired: 9 in, 1 out]
      }
      event "Command Selection": Value Change {
        # "Get the params and show in table"
        n216 = event-data() -> ("NewVal"=w367:i32)  [unwired: 1 in]
        n217 = property on="Command Selection" class="MCListbox (strict)"() -> ("ItemNames"=w365:string[][])  [unwired: 2 in, 2 out]
        n218 = call <vilib>:"WPI_DashboardUpdate Command Params.vi"("NewVal"=w367, "Commands"=w365, "Param Tbl"=w366) -> ()  [unwired: 8 in, 1 out]
      }
      event "Execute Command": Value Change {
        # "Started one, Unique ID holds\nresponse"
        n219 = event-data() -> ()  [unwired: 1 in, 1 out]
        n220 = property on="Command Selection" class="MCListbox (strict)"() -> ("ItemNames"=w379:string[][])  [unwired: 2 in, 2 out]
        n221 = Index Array(array=w379, index (row)="Command Selection", index (col)=0) -> (element=w377:string)
        n222 = call <vilib>:"Invoke Commands.vi"("Command Params"="Command Params", "Function Name"=w377) -> ("Params"=w373:u8, "Started"=w372:bool)  [unwired: 7 in, 1 out]
        n223 = Array Subset(array="Command Params", length (row)=w373) -> (w374:string[][])  [unwired: 3 in]
        n224 = Select(t="Executing" ("Cmd Status"), s=w372, f="" ("Cmd Status")) -> (s? t:f=→"Cmd Status":string)
      }
      event "Command Selection": Double Click {
        n225 = event-data() -> ("Row"=w389:i32)  [unwired: 1 in]
        n226 = property on="Command Selection" class="MCListbox (strict)"() -> ("ItemNames"=w392:string[][])  [unwired: 2 in, 2 out]
        n227 = local read "Command Params"() -> (w387:string[][])
        n228 = Index Array(array=w392, index (row)=w389, index (col)=0) -> (element=w390:string)
        n229 = call <vilib>:"Invoke Commands.vi"("Command Params"=w387, "Function Name"=w390) -> ("Params"=w386:u8, "Started"=w381:bool)  [unwired: 7 in, 1 out]
        n230 = Array Subset(array=w387, length (row)=w386) -> (w385:string[][])  [unwired: 3 in]
        n231 = Select(t="Executing" ("Cmd Status"), s=w381, f="" ("Cmd Status")) -> (s? t:f=w382:string)
        n232 = local write "Cmd Status"(w382) -> ()
      }
      event "CheckList": Double Click {
        # "Shift clears all"
        # "Update symbols on the listbox"
        n233 = event-data() -> ("PlatMods.Shift"=w395:bool, "Row"=w397:i32)  [unwired: 1 in]
        n234 = case shown="True" w395 {
          tunnel: w397 -> [w401 _]
          tunnel: 1 -> [w400 _]
          frame False {
            n235 = property on="CheckList" class="LstBox (strict)"() -> ("Item Symbols"=w399:i32[])  [unwired: 2 in, 2 out]
            n236 = Replace Array Subset(array=w399, new element=w400, index=w401) -> (w398:i32[])
            n237 = property on="CheckList" class="LstBox (strict)"("Item Symbols"=w398) -> ()  [unwired: 2 in, 2 out]
          }
          frame True {
            w402 = 0 ("Top Row")
            n238 = property on="CheckList" class="LstBox (strict)"() -> ("Number of Rows"=w404:u32)  [unwired: 2 in, 2 out]
            n239 = Initialize Array(0, w404) -> (w403:i32[])
            n240 = property on="CheckList" class="LstBox (strict)"("Top Row"=w402, "Value"=w402, "Item Symbols"=w403) -> ()  [unwired: 2 in, 2 out]
          }
        }
      }
      event "CheckList": Key Down {
        # "Update symbols on the listbox\nLeft and right keys check and uncheck"
        n241 = event-data() -> ("VKey"=w409:T23)  [unwired: 1 in]
        n242 = case shown="\"Left\", \"Right\"" w409 {
          selector: w409 -> [w414 _]
          tunnel: eventvkey."Left" ("VKey") -> [w412 _]
          frame "Left", "Right" {
            n243 = Equal?(x=w412, y=w414) -> (x = y?=w413:bool)
            n244 = Select(t=0, s=w413, f=1) -> (s? t:f=w415:i32)
            n245 = property on="CheckList" class="LstBox (strict)"() -> ("Item Symbols"=w418:i32[])  [unwired: 2 in, 2 out]
            n246 = Replace Array Subset(array=w418, new element=w415, index="CheckList") -> (w417:i32[])
            n247 = property on="CheckList" class="LstBox (strict)"("Item Symbols"=w417) -> ()  [unwired: 2 in, 2 out]
          }
          frame Default {
          }
        }
      }
      event "DB Camera Config": Value Change {
        # "Show or hide the cluster of controls, store in ini file"
        n248 = event-data() -> ("NewVal"=w423:bool)  [unwired: 1 in]
        n249 = case shown="False" w423 {
          tunnel: w422 -> [w432 _]
          tunnel: [w425 w443] -> w421
          tunnel: w420 -> [w424 w443]
          frame False {
            w439 = "Camera"
            w442 = FALSE ("Visible")
            n250 = local read "Camera Settings"() -> (w431:T2)
            n251 = Index Array(array=w432) -> (element=w435:cluster{string[]})  [unwired: 1 in]
            n252 = Unbundle(w431) -> ("Frame Rate"=w430:i32, "Compression"=w429:i32, "Size"=w433:u16)
            n253 = Unbundle(w435) -> (w434:string[])
            n254 = Index Array(array=w434, index=w433) -> (element=w428:string)
            n255 = call-poly <vilib>:"Write Key.vi"("section"=w439, "value"=w428, "key"="Size", "refnum"=w424) -> ("refnum out"=w441:T21)  [unwired: 2 in, 5 out]
            n256 = call-poly <vilib>:"Write Key.vi"("section"=w439, "value"=w430, "key"="FrameRate", "refnum"=w441) -> ("refnum out"=w440:T21)  [unwired: 1 in, 6 out]
            n257 = property on="Camera Settings" class="Clust (strict)"("Visible"=w442) -> ()  [unwired: 2 in, 2 out]
            n258 = local write "DB Camera Config"(w442) -> ()
            n259 = call-poly <vilib>:"Write Key.vi"("section"=w439, "value"=w429, "key"="Compression", "refnum"=w440) -> ("refnum out"=w426:T21)  [unwired: 1 in, 6 out]
            n260 = call <vilib>:"Close Config Data.vi"("refnum"=w426) -> ("file path"=w427:path)  [unwired: 2 in, 8 out]
            n261 = call <vilib>:"Open Config Data.vi"("configuration file path"=w427) -> ("refnum"=w425:T21)  [unwired: 8 in, 2 out]
          }
          frame True {
            n262 = property on="Camera Settings" class="Clust (strict)"("Visible"=TRUE) -> ()  [unwired: 2 in, 2 out]
          }
        }
      }
      event "Camera Settings": Value Change {
        # "Update summary string when any elements of DB camera change"
        n263 = event-data() -> ("NewVal"=w457:T2)  [unwired: 1 in]
        n264 = Index Array(array=w453) -> (element=w452:cluster{string[]})  [unwired: 1 in]
        n265 = Unbundle(w457) -> ("Frame Rate"=w448:i32, "Compression"=w447:i32, "Size"=w450:u16)
        n266 = Unbundle(w452) -> (w451:string[])
        n267 = Index Array(array=w451, index=w450) -> (element=w449:string)
        n268 = Format Into String(format string="%s   %dfps   %d%%", w449, w448, w447) -> (resulting string=w454:string)  [unwired: 2 in, 1 out]
        n269 = Build Array(w454) -> (w455:string[])
        n270 = property on="DB Camera Config" class="Bool (strict)"("Strings [4]"=w455) -> ()  [unwired: 2 in, 2 out]
      }
      event "Motor.Enable": Value Change {
        # "When the test mode otor enable helper is set, update that\ntree row item's value"
        n271 = event-data() -> ("NewVal"=w464:bool)  [unwired: 1 in]
        n272 = Unbundle("Motor") -> ("Value"=w463:dbl)  [unwired: 1 out]
        n273 = Select(t=w463, s=w464, f=0.0) -> (s? t:f=w461:dbl)
        n274 = call <vilib>:"NT Write Number.vi"("Numeric"=w461, "Name"=w460) -> ()  [unwired: 9 in, 1 out]
      }
      event "Test Slider": Value Change {
        # "When the test mode slider helper is set, update that\ntree row item's value"
        n275 = event-data() -> ("NewVal"=w468:dbl)  [unwired: 1 in]
        n276 = call <vilib>:"NT Write Number.vi"("Numeric"=w468, "Name"=w469) -> ()  [unwired: 9 in, 1 out]
      }
      event "On/Off": Value Change {
        # "When the test mode on/off helper value is set, update that\ntree row item's value"
        n277 = event-data() -> ("NewVal"=w474:bool)  [unwired: 1 in]
        n278 = Boolean To (0,1)(Boolean=w474) -> (0, 1=w473:i16)
        n279 = call <vilib>:"NT Write Number.vi"("Numeric"=w473, "Name"=w472) -> ()  [unwired: 9 in, 1 out]
      }
      event "Rev/Fwd": Value Change {
        # "When the test mode helper value for relays is set, update that\ntree row item's value"
        n280 = event-data() -> ("NewVal.Forward"=w483:bool, "NewVal.Reverse"=w482:bool)  [unwired: 1 in]
        n281 = Boolean To (0,1)(Boolean=w483) -> (0, 1=w479:i16)
        n282 = Boolean To (0,1)(Boolean=w482) -> (0, 1=w481:i16)
        n283 = Negate(x=w481) -> (-x=w480:i16)
        n284 = Add(x=w479, y=w480) -> (x+y=w478:i16)
        n285 = call <vilib>:"NT Write Number.vi"("Numeric"=w478, "Name"=w477) -> ()  [unwired: 9 in, 1 out]
      }
      event "Test Ring": Value Change {
        # "When a test mode helper value is selected from the ring,\nset the tree item's variable to the string value"
        n286 = event-data() -> ("NewVal"=w488:u16)  [unwired: 1 in]
        n287 = property on="Test Ring" class="Ring (strict)"() -> ("Strings []"=w489:string[])  [unwired: 2 in, 2 out]
        n288 = Index Array(array=w489, index=w488) -> (element=w487:string)
        n289 = call <vilib>:"NT Write String.vi"("String"=w487, "Name"=w486) -> ()  [unwired: 9 in, 1 out]
      }
      event "Rec Mode": Value Change {
        # "Update globals for recording mode and path to read log from.\nClear when logging and let NetworkTables set path for vision to\nuse."
        n290 = event-data() -> ("NewVal"=w501:enum32{"Stop", "Record", "Playback"})  [unwired: 1 in]
        n291 = global write "WPI_DashboardLogging Global.vi" "Logging Filename"(path "") -> ()
        n292 = global write "WPI_DashboardLogging Global.vi" "Recording"(w501) -> ()
        n293 = case shown="\"Playback\"" w501 {
          tunnel: w500 -> [_ w503 w512]
          tunnel: [_ _ w511] -> w497
          tunnel: [_ _ w510] -> _
          tunnel: w495 -> [_ _ w508]
          tunnel: cluster{i32, i32} {-250, 170} -> [_ _ w507]
          tunnel: [_ _ T24 {"Image Size"=TRUE, "Image Type"=TRUE, "Pixel Value"=TRUE, "ROI Information"=TRUE, "Zoom Factor"=FALSE} ("Image Information Shown:All Elements")] -> w493
          tunnel: [_ _ TRUE ("Zoom Factor")] -> w492
          tunnel: w491 -> [_ _ w504]
          frame Default {
          }
          frame "Stop", "Record" {
            # "Place Window too"
            n294 = invoke class="VI" method="FP.Close"(reference=w503) -> (reference out=w502:refnum<vi>)  [unwired: 2 in, 2 out]
            n295 = invoke class="VI" method="Abort VI"(reference=w502) -> ()  [unwired: 2 in, 3 out]
          }
          frame "Playback" {
            n296 = call "Open Playback Panel.vi"("Offset"=w507, "DB VI Ref"=w508, "Playback in"=w512) -> ("Playback out"=w509:refnum<vi>)  [unwired: 8 in]
            n297 = register-events(w509, w504) -> (reference out=w511:refnum<event-registration>, error out=w510:errorcluster)  [unwired: 2 in]
          }
        }
        n298 = property on="Camera Image" class="ImageControl"("Image Information Shown"=w493, "Image Information Visible"=w492) -> ()  [unwired: 2 in, 2 out]
        n299 = call <vilib>:"WPI_DashboardNT Log FieldName Cache.vi"("Operation"=enum16{"Lookup/Add", "Index", "Clear"}."Clear") -> ()  [unwired: 8 in, 3 out]
      }
      event Panel Close {
        w514 = enum32{"Stop", "Record", "Playback"}."Stop" ("Rec Mode")
        # "Playback window has been closed, abort"
        n300 = event-data() -> ()  [unwired: 1 in, 4 out]
        n301 = local write "Rec Mode"(w514) -> ()
        n302 = global write "WPI_DashboardLogging Global.vi" "Recording"(w514) -> ()
      }
      event Panel Close {
        # "Abort playback window and ourself"
        n303 = event-data() -> ()  [unwired: 1 in, 4 out]
        n304 = invoke class="VI" method="FP.Close"(reference=w520) -> (reference out=w519:refnum<vi>)  [unwired: 2 in, 2 out]
        n305 = invoke class="VI" method="Abort VI"(reference=w519) -> (error out=w518:errorcluster)  [unwired: 2 in, 2 out]
        n306 = invoke class="VI" method="Abort VI"(error in=w518) -> ()  [unwired: 2 in, 3 out]
      }
      event User Event {
        n307 = event-data() -> ("IDs"=w528:cluster{"RPC field ID":u16, "Unique ID":u16}, "String"=w527:string)  [unwired: 1 in]
        n308 = Bundle("IDs"=w528, "String"=w527) -> (w526:T10)  [unwired: 1 in]
        n309 = call <vilib>:"Retrieve RPC Response.vi"("RPC Response"=w526) -> ("Output"=w523:string[][])  [unwired: 10 in]
        n310 = Build Array (concatenate)(w521, w523) -> (w522:string[][])
        n311 = local write "Command Params"(w522) -> ()
        n312 = local write "Cmd Status"("" ("Cmd Status")) -> ()
      }
      event "Vision": Value Change {
        # "Enable/Disable Compression slider.\nHW USB is hard-coded into the camera"
        n313 = event-data() -> ("NewVal"=w535:u16)  [unwired: 1 in]
        n314 = Equal?(x=w535, y=u32 2 ("milliseconds to wait")) -> (x = y?=w533:bool)
        n315 = Select(t=T25."Disabled and Grayed Out" ("Disabled"), s=w533, f=T25."Enabled" ("Disabled")) -> (s? t:f=w530:T25)
        n316 = property on="Compression" class="Slide (strict)"("DisabledEnum"=w530) -> ()  [unwired: 2 in, 2 out]
      }
      event "Tree": Double Click {
        n317 = event-data() -> ("PlatMods"=w540:T28, "Tag"=w539:string)  [unwired: 1 in]
        n318 = Unbundle(w540) -> ("Shift"=w538:bool)  [unwired: 4 out]
        n319 = Not(x=w538) -> (.not. x?=w537:bool)
        n320 = call <vilib>:"NT Update Persistence.vi"("Persistence"=w537, "Name"=w539) -> ()  [unwired: 9 in, 1 out]
      }
    }
  }
  n321 = while {
    tunnel: w45 -> [w546]
    i -> [w549]
    stop <- FALSE stop-if-true
    n322 = local read "Mode"() -> (w544:T6)
    n323 = Tick Count (ms)() -> (millisecond timer value=w543:u32)
    n324 = Wait (ms)(milliseconds to wait=u32 100) -> ()  [unwired: 1 out]
    n325 = case shown="\"Stop\", Default" "Rec Mode" {
      tunnel: w549 -> [_ _ w564]
      tunnel: [u32 0 u32 11141120 ("Target Color") w553] -> w545
      tunnel: w544 -> [_ _ _]
      tunnel: w543 -> [_ _ _]
      frame "Stop", Default {
      }
      frame "Record" {
      }
      frame "Playback" {
        # "Playback"
        n326 = Quotient & Remainder(x=w564, y=u32 50 ("milliseconds to wait")) -> (x-y*floor(x/y)=w560:u32)  [unwired: 1 out]
        n327 = Divide(x=w560, y=u32 50 ("milliseconds to wait")) -> (x/y=w557:dbl)
        n328 = Multiply(x=6.283185307179586, y=w557) -> (x*y=w562:dbl)
        n329 = Sine(x=w562) -> (sin(x)=w561:dbl)
        n330 = Absolute Value(x=w561) -> (abs(x)=w554:dbl)
        n331 = call "Interpolate RGB Color.vi"("Proportion"=w554, "Target Color"=u32 30976, "Base Color"=u32 2829099) -> ("Result Color"=w553:u32)  [unwired: 8 in]
      }
    }
    n332 = property class="Pane"(reference=w546, "PaneColor"=w545) -> ()  [unwired: 1 in, 2 out]
  }
  n333 = local write "Dashboard Tab"(T1."Drive" ("Dashboard Tab")) -> ()
  n334 = property on="On/Off" class="Bool (strict)"("Visible"=w15) -> ()  [unwired: 2 in, 2 out]
  n335 = property on="Motor" class="Clust (strict)"("Visible"=w15) -> ()  [unwired: 2 in, 2 out]
  n336 = property on="Progress" class="Clust (strict)"("Visible"=w15) -> ()  [unwired: 2 in, 2 out]
  n337 = property on="Test Ring" class="Ring (strict)"("Visible"=w15) -> ()  [unwired: 2 in, 2 out]
  n338 = property on="Rev/Fwd" class="Clust (strict)"("Visible"=w15) -> ()  [unwired: 2 in, 2 out]
  n339 = property on="Camera Settings" class="Clust (strict)"("Visible"=w15) -> ()  [unwired: 2 in, 2 out]
  n340 = while {
    tunnel: u16 1741 ("timeout ms (25000)") -> [w566]
    stop <- FALSE stop-if-true
    n341 = TCP Create Listener(10:w566) -> (0:w565:errorcluster, 3:w567:refnum<k5>)  [unwired: 4 in, 1 out]
    n342 = case shown="No Error" w565 {
      selector: w565 -> [w569 _]
      tunnel: w567 -> [w570 _]
      frame No Error {
        n343 = while {
          tunnel: w570 -> [w573]
          tunnel: w569 -> [w572]
          stop <- FALSE stop-if-true
          n344 = TCP Wait On Listener(8:w572, 11:w573) -> (0:w574:errorcluster, 4:w575:refnum<k5>)  [unwired: 2 in, 3 out]
          n345 = local write "TCP"(w575) -> ()
          n346 = case shown="No Error" w574 {
            frame No Error {
            }
            frame Error {
              n347 = Wait (ms)(milliseconds to wait=u32 1000) -> ()  [unwired: 1 out]
            }
          }
        }
      }
      frame Error {
        n348 = Wait (ms)(milliseconds to wait=u32 1000) -> ()  [unwired: 1 out]
      }
    }
  }
  n349 = local write "DB Camera Config"(w15) -> ()
  n350 = local write "Command Params"(string[][] [] ("Command Params")) -> ()
  n351 = global write "WPI_DashboardLogging Global.vi" "Recording"(w39) -> ()
  n352 = local write "Command Selection"(u16 0 ("milliseconds to wait")) -> ()
  n353 = local write "Rec Mode"(w39) -> ()
